vi "Voltage-Selection.vi"(0 "ESTOP":bool, 5 "VFD \nMode\nSelect":bool, 9 "PID In":dbl, 12 "Percentage\nIn":dbl) -> (4 "output":dbl)   [LabVIEW 2025]
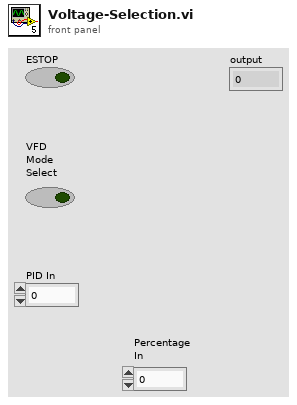
[diagram p1: front panel]
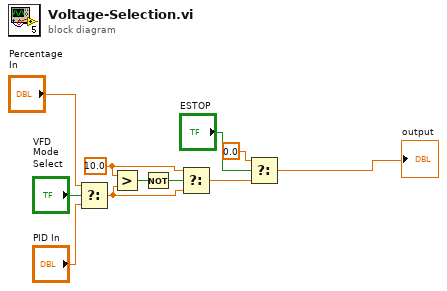
[diagram p0: block diagram]
diagram:
  w5 = 10.0 ("x")
  n1 = Select(t="Percentage\nIn", s="VFD \nMode\nSelect", f="PID In") -> (s? t:f=w4:dbl)
  n2 = Greater?(x=w5, y=w4) -> (0:w8:bool)
  n3 = Not(x=w8) -> (.not. x?=w9:bool)
  n4 = Select(t=w5, s=w9, f=w4) -> (s? t:f=w7:dbl)
  n5 = Select(t=0.0, s="ESTOP", f=w7) -> (s? t:f=→"output":dbl)
